vi "Set_Panel_Scaling_for_Page.vi"(2 "error in":errorcluster, 3 "panel scaling for page (unchanged)":T1 items=["Unchanged", "No Scaling", "Scale front panel to fit"], 4 "VI Refnum":refnum<vi>) -> (0 "error out":errorcluster, 1 "VI Refnum out":refnum<vi>)   [LabVIEW 2017, in "NI_ReportGenerationCore.lvlib"]
uses:
  <vilib>/Utility/NIReport.llb/NI_ReportGenerationCore.lvlib
  <vilib>/printing/EasyPrintingControls.llb/panel_scaling_for_page.ctl
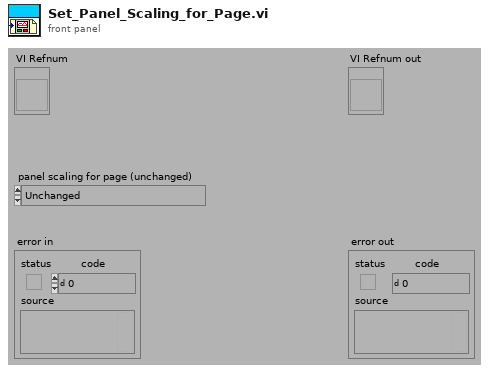
[diagram p1: front panel]
types:
  T1 = typedef "NI_ReportGenerationCore.lvlib/panel_scaling_for_page.ctl" = u16
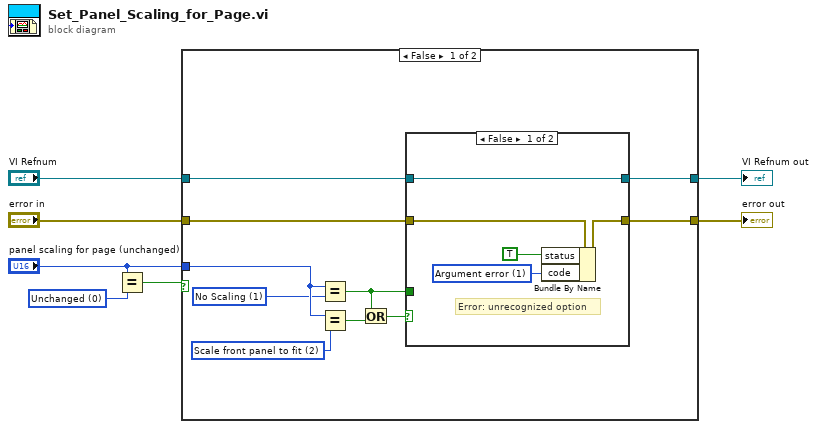
[diagram p0: block diagram]
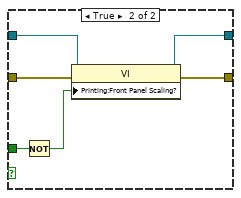
[diagram p2: hidden frame]
diagram:
  w2 = T1 0 items=["Unchanged", "No Scaling", "Scale down to page", "Scale up to page", "Fit to Page"] ("panel scaling for page (unchanged)")
  n1 = Equal?(x="panel scaling for page (unchanged)", y=w2) -> (x = y?=w4:bool)
  n2 = case shown="False" w4 {
    tunnel: "panel scaling for page (unchanged)" -> [w11 _]
    tunnel: "VI Refnum" -> [w14 w30]
    tunnel: "error in" -> [w16 w29]
    tunnel: [w15 w29] -> w7
    tunnel: [w13 w30] -> w3
    frame False {
      w8 = T1 2 items=["Unchanged", "No Scaling", "Scale front panel to fit"] ("panel scaling for page (unchanged)")
      w9 = T1 1 items=["Unchanged", "No Scaling", "Scale front panel to fit"] ("panel scaling for page (unchanged)")
      n3 = Equal?(x=w11, y=w9) -> (x = y?=w12:bool)
      n4 = Equal?(x=w11, y=w8) -> (x = y?=w10:bool)
      n5 = Or(x=w12, y=w10) -> (x .or. y?=w17:bool)
      n6 = case shown="False" w17 {
        tunnel: w16 -> [w20 w27]
        tunnel: [w18 w26] -> w15
        tunnel: w14 -> [w19 w28]
        tunnel: [w19 w23] -> w13
        tunnel: w12 -> [_ w24]
        frame False {
          w21 = 1 items=["No error", "Argument error", "Memory is full", "Out of zone", "End of file", "File already open", "Generic file I/O error", "File not found", "File permission error", "Disk is full", "Duplicate path", "Too many files open", "System feature not enabled", "Resource file not found", "Cannot add resource", "Resource not found", "Image not found", "Image memory error", "Pen does not exist", "Config type invalid", "Config token not found", "Config parse error", "Config memory error", "Bad external code format", "Bad external code offset", "External code not present", "Null window", "Destroy window error", "Null menu", "Print aborted", "Bad print record", "Print driver error", "Windows error during printing", "Memory error during printing", "Print dialog error", "Generic print error", "Invalid device refnum", "Device not found", "Device parameter error", "Device unit error", "Cannot open device", "Device call aborted", "Generic error", "Cancelled by user", "Object ID too low", "Object ID too high", "Object not in heap", "Unknown heap", "Unknown object (invalid DefProc)", "Unknown object (DefProc not in table)", "Message out of range", "Invalid (null) method", "Unknown message", "Manager call not supported", "Bad address", "Network operation in progress", "Network operation timed out", "Connection is busy", "Network attribute not supported", "Network error", "Address in use", "System out of memory", "Connection aborted", "Connection refused", "Not connected", "Already connected", "Connection closed", "Initialization error (interapplication manager)", "Bad occurrence", "Wait on unbound occurrence handler", "Occurrence queue overflow", "Datalog type conflict", "Unused", "Unrecognized type (interapplication manager)", "Memory corrupt", "Failed to make temporary DLL", "Old CIN version", "Drag socket not found", "Failed to load drop-object", "Failed to register OLE object", "Failed to release OLE object", "Format specifier type mismatch", "Unknown format specifier", "Too few format specifiers", "Too many format specifiers", "Scan failed", "Newer CIN version", "Error converting to variant", "Runtime menu error", "Password tampered", "Variant attribute not found", "Incompatible variant data type", "Event data is not available", "Event Store is not present", "Occurrence is not found", "Event Queue is not created", "Event info is not available", "Refnum passed is NULL", "Error retrieving Class GUID", "Error retrieving CoClass GUID", "Error retrieving TypeLib GUID.", "Bad built application magic bytes.", "Specific driver is different from the specific driver associated with the Logical Name.", "There is no session opened to the class driver.", "Max Error", "MAX - Error with config objects", "MAX - Error loading configuration", "MAX - Group not supported"]
          # "Error: unrecognized option"
          n7 = Bundle By Name(cluster=w20, "status"=TRUE, "code"=w21) -> (w18:errorcluster)
        }
        frame True {
          n8 = Not(x=w24) -> (.not. x?=w25:bool)
          n9 = property class="VI"(reference=w28, error in=w27, "Printing:Front Panel Scaling?"=w25) -> (reference out=w23:refnum<vi>, error out=w26:errorcluster)
        }
      }
    }
    frame True {
      # "Do not change this setting"
    }
  }
  "VI Refnum out" <- w3
  "error out" <- w7
